vi "REQ Channel Setting.vi"(8 "error in":errorcluster, 10 "Channel Setting":T1={"Channel Name (0: Channel 1)"=0, "Coupling (1: DC)"=1, "Vertical Offset (0.0)"=0.0, "Vertical Range (40.0 V)"=40.0, "Probe Attenuation (1.0)"=1.0, "Enable Channel (T: Enable)"=TRUE, "Impedance (0: 1 MOhm)"=0, "Vertical Scale (5.0 V)"=5.0, "Vertical Setting (1: Vertical Range)"=1} {"Vertical Setting (1: Vertical Range)" items=["Vertical Scale", "Vertical Range"]; "Impedance (0: 1 MOhm)" items=["1 MOhm", "50 Ohm"]; "Coupling (1: DC)" items=["AC", "DC"]; "Channel Name (0: Channel 1)" items=["Channel 1", "Channel 2", "Channel 3", "Channel 4"]}) -> (0 "error out":errorcluster)   [LabVIEW 2021, in "Oscilloscope.lvlib"]
doc: "_____\nCreated using DQMH Event Scripter 6.1.0.128."
uses:
  Oscilloscope.lvlib
  REQ Channel Setting Argument--cluster.ctl
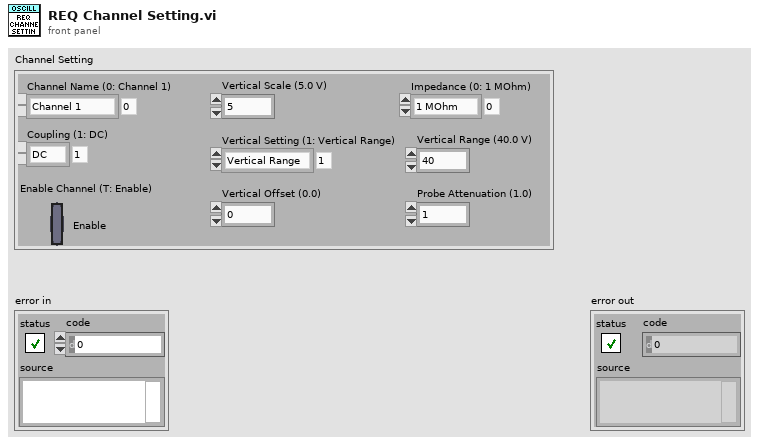
[diagram p1: front panel]
types:
  T1 = cluster{"Channel Name (0: Channel 1)":i32, "Coupling (1: DC)":i32, "Vertical Offset (0.0)":dbl, "Vertical Range (40.0 V)":dbl, "Probe Attenuation (1.0)":dbl, "Enable Channel (T: Enable)":bool, "Impedance (0: 1 MOhm)":i32, "Vertical Scale (5.0 V)":dbl, "Vertical Setting (1: Vertical Range)":i32}
  T2 = typedef "Oscilloscope.lvlib/REQ Channel Setting Argument--cluster.ctl" = cluster{"Channel Setting":cluster{"Channel Name (0: Channel 1)":i32, "Coupling (1: DC)":i32, "Vertical Offset (0.0)":dbl, "Vertical Range (40.0 V)":dbl, "Probe Attenuation (1.0)":dbl, "Enable Channel (T: Enable)":bool, "Impedance (0: 1 MOhm)":i32, "Vertical Scale (5.0 V)":dbl, "Vertical Setting (1: Vertical Range)":i32}}
  T3 = typedef "Oscilloscope.lvlib/Request Events--cluster.ctl" = cluster{"Stop Module":refnum<user-event>, "Show Panel":refnum<user-event>, "Hide Panel":refnum<user-event>, "Get Module Execution Status":refnum<user-event>, "Show Diagram":refnum<user-event>, "REQ Initialize Hardware":refnum<user-event>, "REQ Auto setup":refnum<user-event>, "Close Ref":refnum<user-event>, "Acquire Waveform":refnum<user-event>, "REQ Channel Setting":refnum<user-event>, "REQ Configure DVM":refnum<user-event>, "REQ Read DVM":refnum<user-event>}
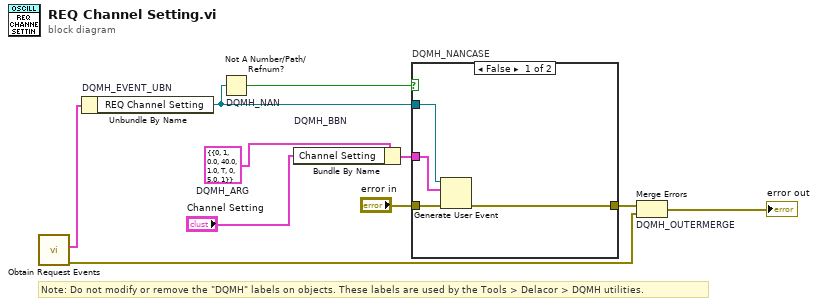
[diagram p0: block diagram]
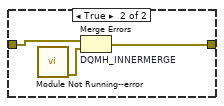
[diagram p2: hidden frame]
diagram:
  w4 = T2 {"Channel Setting"={"Channel Name (0: Channel 1)"=0, "Coupling (1: DC)"=1, "Vertical Offset (0.0)"=0.0, "Vertical Range (40.0 V)"=40.0, "Probe Attenuation (1.0)"=1.0, "Enable Channel (T: Enable)"=TRUE, "Impedance (0: 1 MOhm)"=0, "Vertical Scale (5.0 V)"=5.0, "Vertical Setting (1: Vertical Range)"=1}}  # DQMH_ARG
  # "Note: Do not modify or remove the \"DQMH\" labels on objects. These labels are used by the Tools > Delacor > DQMH utilities."
  n1 = call "Obtain Request Events.vi"() -> ("error out"=w2:errorcluster, "Oscilloscope Request Events"=w1:T3)  [unwired: 10 in]
  n2 = Unbundle By Name "DQMH_EVENT_UBN"(w1) -> ("REQ Channel Setting"=w6:refnum<user-event>)
  n3 = Not A Number/Path/Refnum? "DQMH_NAN"(number/path/refnum=w6) -> (NaN/Path/Refnum?=w7:bool)
  n4 = Bundle By Name "DQMH_BBN"(cluster=w4, "Channel Setting"="Channel Setting") -> (w8:T2)
  n5 = case "DQMH_NANCASE" shown="False" w7 {
    tunnel: "error in" -> [w14 w17]
    tunnel: [w13 w16] -> w5
    tunnel: w6 -> [w12 _]
    tunnel: w8 -> [w11 _]
    frame False {
      n6 = Generate User Event(user event=w12, event data cluster=w11, error in=w14) -> (error out=w13:errorcluster)  [unwired: 1 in, 1 out]
    }
    frame True {
      n7 = call "Module Not Running--error.vi"() -> ("error out"=w15:errorcluster)  [unwired: 11 in]
      n8 = Merge Errors "DQMH_INNERMERGE"(w17, w15) -> (w16:errorcluster)
    }
  }
  n9 = Merge Errors "DQMH_OUTERMERGE"(w5, w2) -> (→"error out":errorcluster)
